vi "Update Bind RPC Template.vi"(8 "error in (no error)":errorcluster, 11 "Server Library (Library Item) in":refnum<vi>) -> (0 "error out":errorcluster, 3 "Server Library (Library Item) out":refnum<vi>)   [LabVIEW 2019, in "gRPC Template Creation Utility.lvlib"]
uses:
  gRPC Template Creation Utility.lvlib
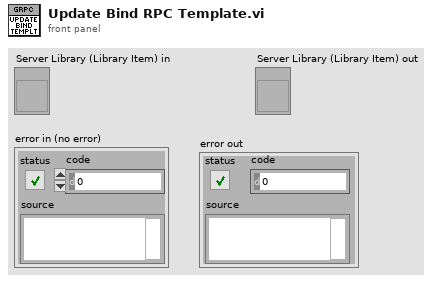
[diagram p1: front panel]
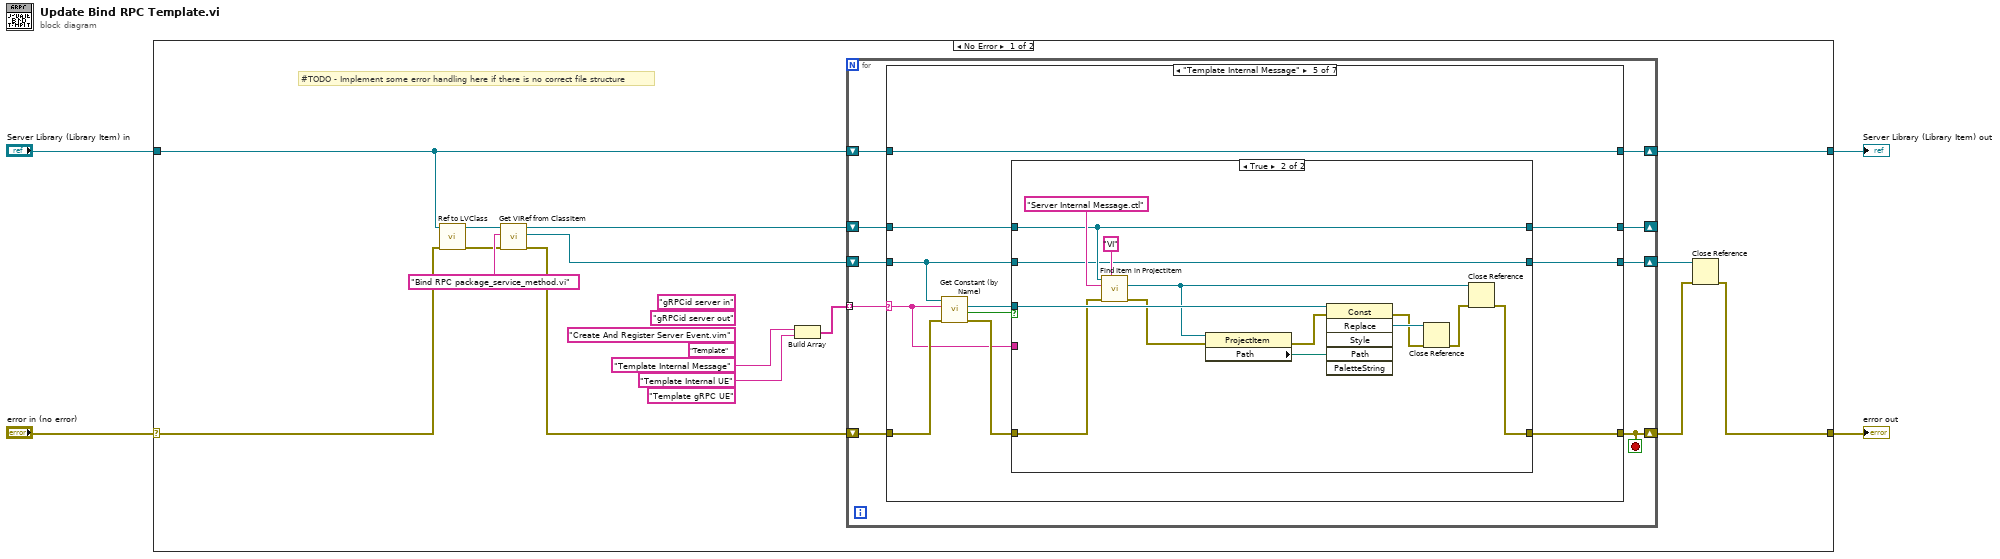
[diagram p0: block diagram]
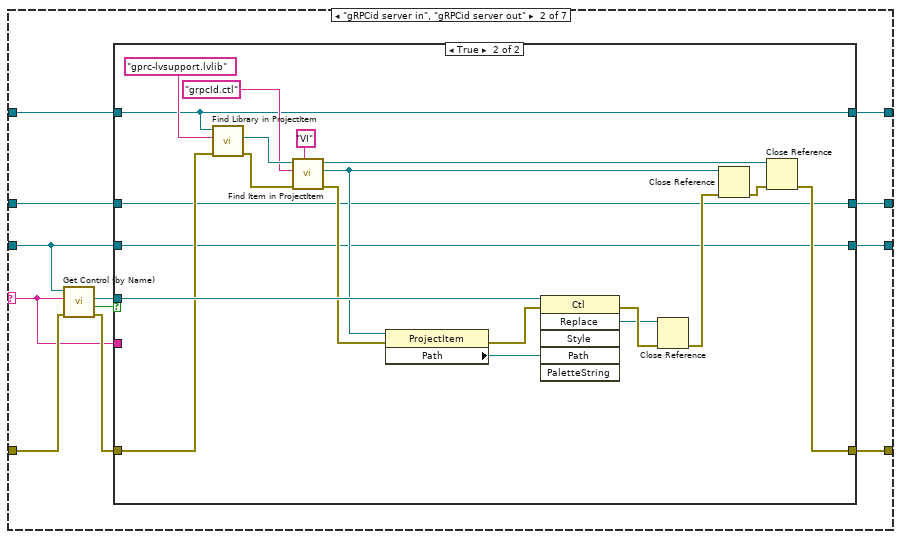
[diagram p3: hidden frame]
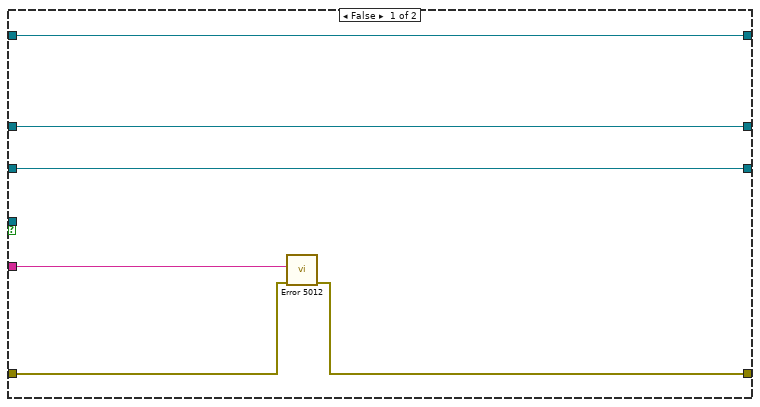
[diagram p4: hidden frame]
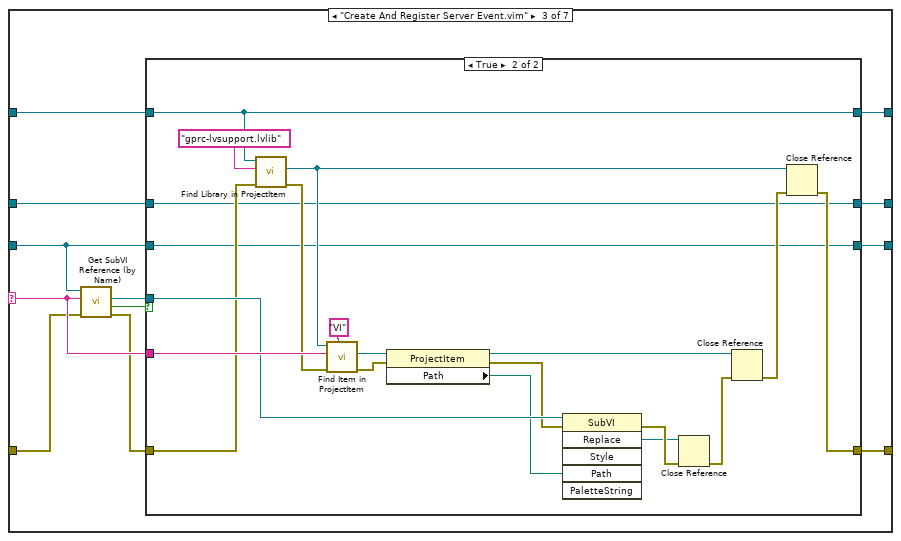
[diagram p5: hidden frame]
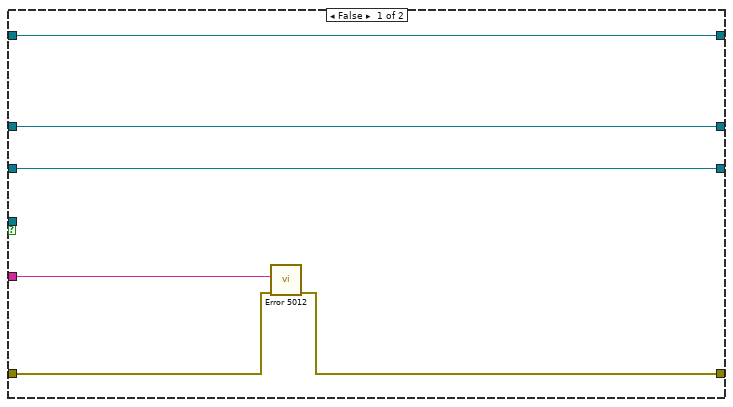
[diagram p6: hidden frame]
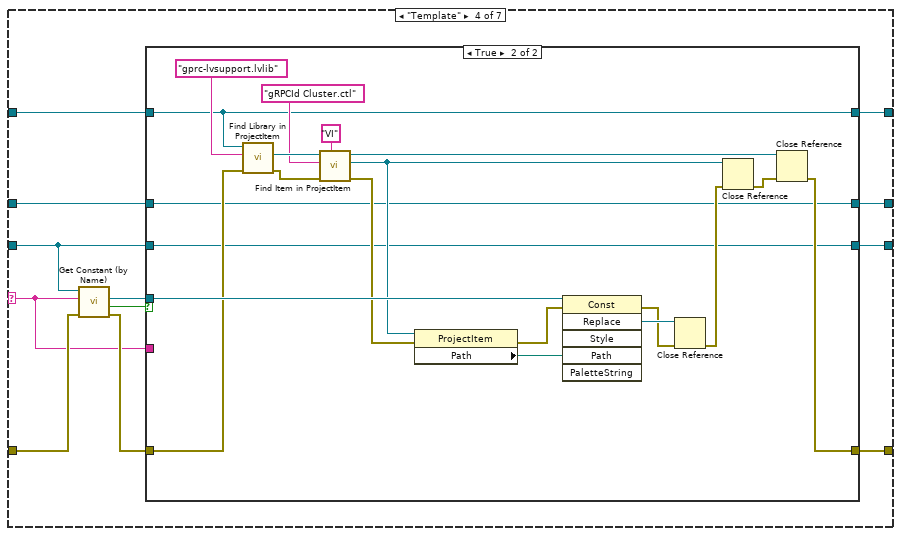
[diagram p7: hidden frame]
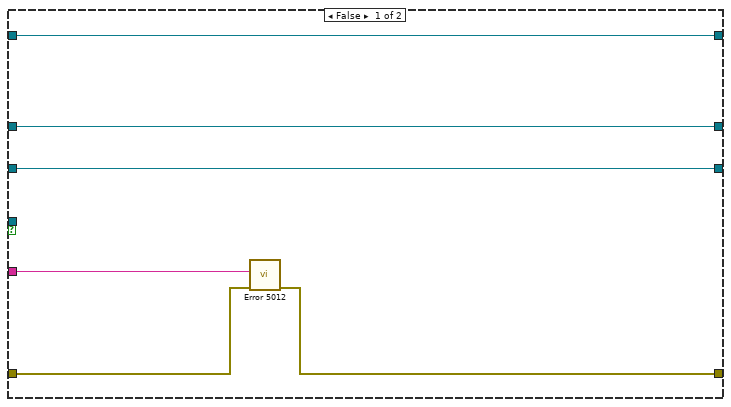
[diagram p8: hidden frame]
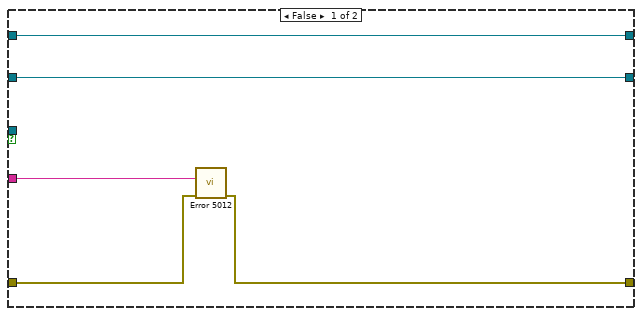
[diagram p9: hidden frame]
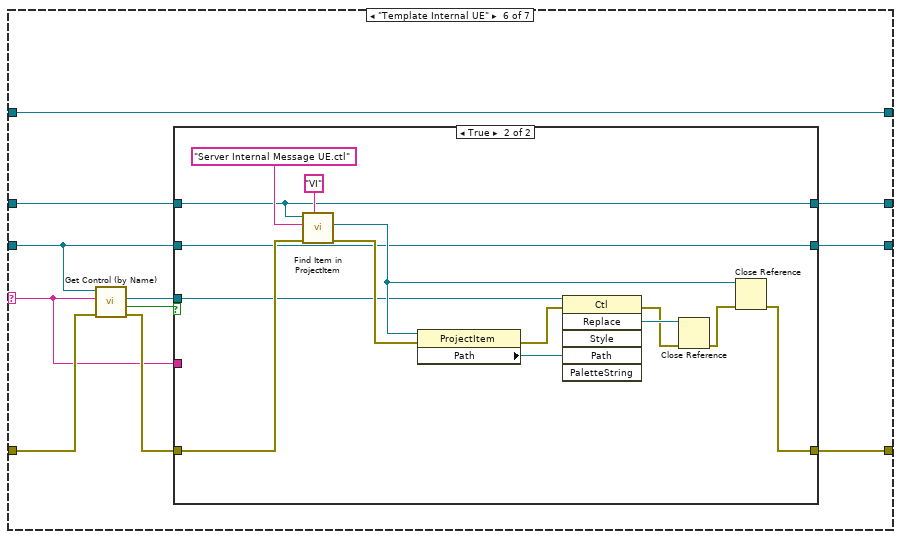
[diagram p10: hidden frame]
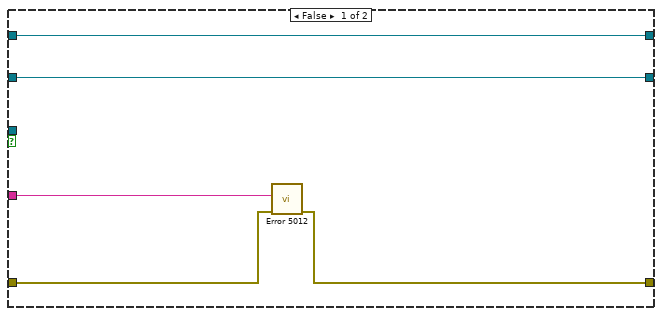
[diagram p11: hidden frame]
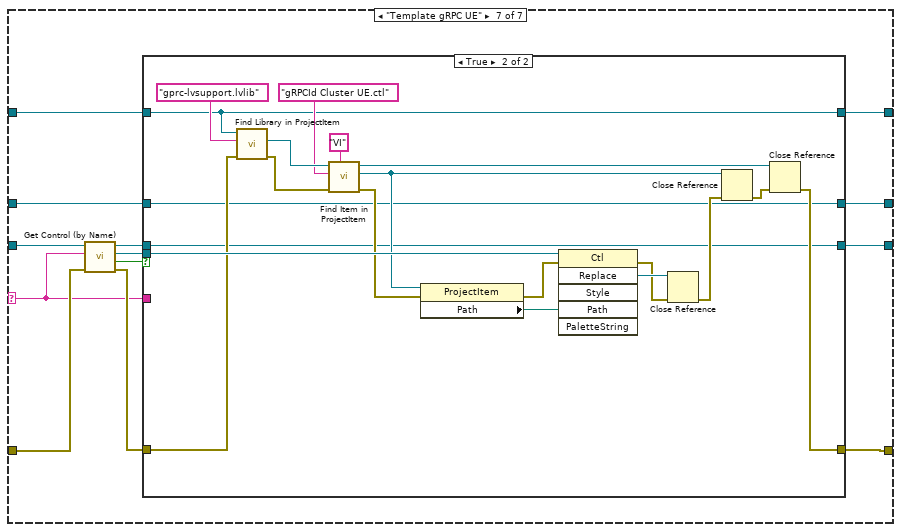
[diagram p12: hidden frame]
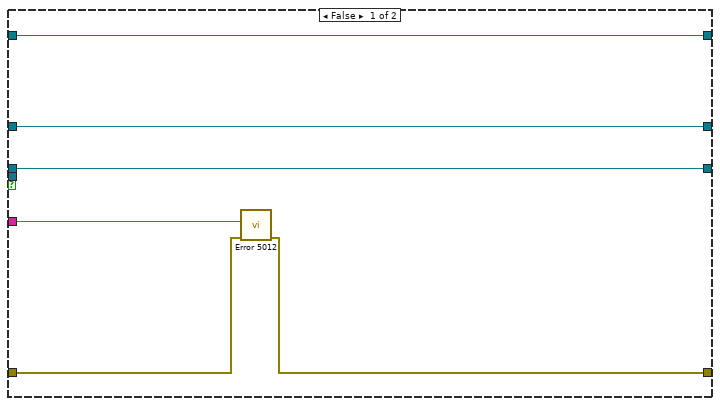
[diagram p13: hidden frame]
diagram:
  n1 = case shown="No Error" "error in (no error)" {
    selector: "error in (no error)" -> [w18 w247]
    tunnel: "Server Library (Library Item) in" -> [w5 w246]
    tunnel: [w8 w247] -> w3
    tunnel: [w11 w246] -> w1
    frame No Error {
      (unwired) "Template gRPC UE" ("Item Name")
      (unwired) "Template" ("Item Name")
      (unwired) "Create And Register Server Event.vim" ("Item Name")
      (unwired) "gRPCid server out" ("Item Name")
      (unwired) "gRPCid server in" ("Item Name")
      # "#TODO - Implement some error handling here if there is no correct file structure"
      n2 = call "Ref to LVClass.vi"("error in (no error)"=w18, "ProjectItem in"=w5) -> ("error out"=w6:errorcluster, "LVClassLibrary out"=w7:refnum<vi>)  [unwired: 8 in]
      n3 = call "Get VIRef from ClassItem.vi"("error in (no error)"=w6, "Item Name"="Bind RPC package_service_method.vi", "LVClassLibrary in"=w7) -> ("error out"=w13:errorcluster, "VIref out"=w12:refnum<vi>, "LVClassLibrary out"=w15:refnum<vi>)  [unwired: 5 in, 1 out]
      n4 = Build Array("Template Internal Message" ("Item Name"), "Template Internal UE" ("Item Name")) -> (w14:string[])
      n5 = for {
        shift-right: [w26] -> w11
        shift-left: w5 -> [w27]
        tunnel: w14 -> [w28] mode=indexing
        shift-right: [w20] -> w9
        shift-left: w13 -> [w25]
        shift-right: [w22] -> _
        shift-left: w15 -> [w23]
        shift-right: [w21] -> w10
        shift-left: w12 -> [w24]
        stop <- w20 stop-if-true
        n6 = case shown="\"Template Internal Message\"" w28 {
          selector: w28 -> [_ w33 w81 w109 w147 w177 w207]
          tunnel: w27 -> [w32 w44 w82 w120 w157 w187 w216]
          tunnel: [w32 w34 w71 w110 w157 w187 w212] -> w26
          tunnel: w24 -> [w29 w38 w75 w114 w149 w180 w219]
          tunnel: w25 -> [w31 w42 w79 w118 w155 w185 w218]
          tunnel: [w31 w40 w77 w116 w154 w186 w214] -> w20
          tunnel: w23 -> [w30 w36 w73 w112 w152 w182 w211]
          tunnel: [w30 w35 w72 w111 w150 w178 w210] -> w22
          tunnel: [w29 w37 w74 w113 w148 w179 w208] -> w21
          frame "None", Default {
          }
          frame "gRPCid server in", "gRPCid server out" {
            n7 = call "Get Control (by Name).vi"("error in (no error)"=w42, "Control Label"=w33, "Owner VI in"=w38) -> ("error out"=w41:errorcluster, "Found ?"=w39:bool, "Control Refnum"=w43:refnum<vi>)  [unwired: 5 in, 1 out]
            n8 = case shown="True" w39 {
              tunnel: w44 -> [w50 w51]
              tunnel: w43 -> [_ w66]
              tunnel: w41 -> [w47 w64]
              tunnel: [w45 w54] -> w40
              tunnel: w38 -> [w48 w53]
              tunnel: [w48 w53] -> w37
              tunnel: w36 -> [w49 w52]
              tunnel: [w49 w52] -> w35
              tunnel: [w50 w51] -> w34
              tunnel: w33 -> [w46 _]
              frame False {
                n9 = call "Error 5012.vi"("error in (no error)"=w47, "Element Name"=w46) -> ("error out"=w45:errorcluster)  [unwired: 9 in]
              }
              frame True {
                n10 = call "Find Library in ProjectItem.vi"("error in (no error)"=w64, "Library Name"="gprc-lvsupport.lvlib", "ProjectItem in"=w51) -> ("error out"=w63:errorcluster, "Library out"=w69:refnum<vi>)  [unwired: 5 in, 2 out]
                n11 = call "Find Item in ProjectItem.vi"("Item Type"="VI", "error in (no error)"=w63, "Name"="grpcId.ctl", "ProjectItem in"=w69) -> ("error out"=w62:errorcluster, "Item Refnum out"=w57:refnum<vi>, "ProjectItem out"=w55:refnum<vi>)  [unwired: 4 in, 1 out]
                n12 = property class="ProjectItem"(reference=w57, error in=w62) -> (error out=w59:errorcluster, "Path"=w65:path)  [unwired: 1 out]
                n13 = invoke class="Ctl" method="Replace"(reference=w66, error in=w59, "Path"=w65) -> (error out=w61:errorcluster, "Replace"=w60:refnum<vi>)  [unwired: 3 in, 4 out]
                n14 = Close Reference(reference=w60, error in (no error)=w61) -> (error out=w58:errorcluster)
                n15 = Close Reference(reference=w57, error in (no error)=w58) -> (error out=w56:errorcluster)
                n16 = Close Reference(reference=w55, error in (no error)=w56) -> (error out=w54:errorcluster)
              }
            }
          }
          frame "Create And Register Server Event.vim" {
            n17 = call "Get SubVI Reference (by Name).vi"("error in (no error)"=w79, "SubVI Name"=w81, "Owner VI in"=w75) -> ("error out"=w78:errorcluster, "Found ?"=w76:bool, "SubVI Refnum out"=w80:refnum<vi>)  [unwired: 5 in, 1 out]
            n18 = case shown="True" w76 {
              tunnel: w82 -> [w88 w89]
              tunnel: w81 -> [w84 w106]
              tunnel: w80 -> [_ w105]
              tunnel: w78 -> [w85 w100]
              tunnel: [w83 w92] -> w77
              tunnel: w75 -> [w86 w91]
              tunnel: [w86 w91] -> w74
              tunnel: w73 -> [w87 w90]
              tunnel: [w87 w90] -> w72
              tunnel: [w88 w89] -> w71
              frame False {
                n19 = call "Error 5012.vi"("error in (no error)"=w85, "Element Name"=w84) -> ("error out"=w83:errorcluster)  [unwired: 9 in]
              }
              frame True {
                n20 = call "Find Library in ProjectItem.vi"("error in (no error)"=w100, "Library Name"="gprc-lvsupport.lvlib", "ProjectItem in"=w89) -> ("error out"=w99:errorcluster, "Library out"=w94:refnum<vi>)  [unwired: 5 in, 2 out]
                n21 = call "Find Item in ProjectItem.vi"("Item Type"="VI", "error in (no error)"=w99, "Name"=w106, "ProjectItem in"=w94) -> ("error out"=w98:errorcluster, "Item Refnum out"=w104:refnum<vi>)  [unwired: 4 in, 2 out]
                n22 = property class="ProjectItem"(reference=w104, error in=w98) -> (reference out=w96:refnum<vi>, error out=w97:errorcluster, "Path"=w103:path)
                n23 = invoke class="SubVI" method="Replace"(reference=w105, error in=w97, "Path"=w103) -> (error out=w102:errorcluster, "Replace"=w101:refnum<vi>)  [unwired: 3 in, 4 out]
                n24 = Close Reference(reference=w101, error in (no error)=w102) -> (error out=w95:errorcluster)
                n25 = Close Reference(reference=w96, error in (no error)=w95) -> (error out=w93:errorcluster)
                n26 = Close Reference(reference=w94, error in (no error)=w93) -> (error out=w92:errorcluster)
              }
            }
          }
          frame "Template" {
            n27 = call "Get Constant (by Name).vi"("error in (no error)"=w118, "Constant Label"=w109, "Owner VI in"=w114) -> ("error out"=w117:errorcluster, "Found ?"=w115:bool, "Const ref out"=w119:refnum<vi>)  [unwired: 5 in, 1 out]
            n28 = case shown="True" w115 {
              tunnel: w120 -> [w126 w127]
              tunnel: w119 -> [_ w140]
              tunnel: w117 -> [w122 w133]
              tunnel: [w121 w130] -> w116
              tunnel: w114 -> [w124 w129]
              tunnel: [w124 w129] -> w113
              tunnel: w112 -> [w125 w128]
              tunnel: [w125 w128] -> w111
              tunnel: [w126 w127] -> w110
              tunnel: w109 -> [w123 _]
              frame False {
                n29 = call "Error 5012.vi"("error in (no error)"=w122, "Element Name"=w123) -> ("error out"=w121:errorcluster)  [unwired: 9 in]
              }
              frame True {
                n30 = call "Find Library in ProjectItem.vi"("error in (no error)"=w133, "Library Name"="gprc-lvsupport.lvlib", "ProjectItem in"=w127) -> ("error out"=w132:errorcluster, "Library out"=w145:refnum<vi>)  [unwired: 5 in, 2 out]
                n31 = call "Find Item in ProjectItem.vi"("Item Type"="VI", "error in (no error)"=w132, "Name"="gRPCId Cluster.ctl", "ProjectItem in"=w145) -> ("error out"=w131:errorcluster, "Item Refnum out"=w137:refnum<vi>, "ProjectItem out"=w135:refnum<vi>)  [unwired: 4 in, 1 out]
                n32 = property class="ProjectItem"(reference=w137, error in=w131) -> (error out=w141:errorcluster, "Path"=w142:path)  [unwired: 1 out]
                n33 = invoke class="Const" method="Replace"(reference=w140, error in=w141, "Path"=w142) -> (error out=w138:errorcluster, "Replace"=w139:refnum<vi>)  [unwired: 3 in, 4 out]
                n34 = Close Reference(reference=w139, error in (no error)=w138) -> (error out=w136:errorcluster)
                n35 = Close Reference(reference=w137, error in (no error)=w136) -> (error out=w134:errorcluster)
                n36 = Close Reference(reference=w135, error in (no error)=w134) -> (error out=w130:errorcluster)
              }
            }
          }
          frame "Template Internal Message" {
            n37 = call "Get Constant (by Name).vi"("error in (no error)"=w155, "Constant Label"=w147, "Owner VI in"=w149) -> ("error out"=w153:errorcluster, "Found ?"=w151:bool, "Const ref out"=w156:refnum<vi>)  [unwired: 5 in, 1 out]
            n38 = case shown="True" w151 {
              tunnel: w156 -> [_ w172]
              tunnel: [w158 w166] -> w154
              tunnel: w153 -> [w159 w165]
              tunnel: w152 -> [w162 w164]
              tunnel: [w162 w164] -> w150
              tunnel: w149 -> [w161 w163]
              tunnel: [w161 w163] -> w148
              tunnel: w147 -> [w160 _]
              frame False {
                n39 = call "Error 5012.vi"("error in (no error)"=w159, "Element Name"=w160) -> ("error out"=w158:errorcluster)  [unwired: 9 in]
              }
              frame True {
                n40 = call "Find Item in ProjectItem.vi"("Item Type"="VI", "error in (no error)"=w165, "Name"="Server Internal Message.ctl", "ProjectItem in"=w164) -> ("error out"=w167:errorcluster, "Item Refnum out"=w169:refnum<vi>)  [unwired: 4 in, 2 out]
                n41 = property class="ProjectItem"(reference=w169, error in=w167) -> (error out=w173:errorcluster, "Path"=w174:path)  [unwired: 1 out]
                n42 = invoke class="Const" method="Replace"(reference=w172, error in=w173, "Path"=w174) -> (error out=w170:errorcluster, "Replace"=w171:refnum<vi>)  [unwired: 3 in, 4 out]
                n43 = Close Reference(reference=w171, error in (no error)=w170) -> (error out=w168:errorcluster)
                n44 = Close Reference(reference=w169, error in (no error)=w168) -> (error out=w166:errorcluster)
              }
            }
          }
          frame "Template Internal UE" {
            n45 = call "Get Control (by Name).vi"("error in (no error)"=w185, "Control Label"=w177, "Owner VI in"=w180) -> ("error out"=w184:errorcluster, "Found ?"=w181:bool, "Control Refnum"=w183:refnum<vi>)  [unwired: 5 in, 1 out]
            n46 = case shown="True" w181 {
              tunnel: [w189 w197] -> w186
              tunnel: w184 -> [w190 w196]
              tunnel: w183 -> [_ w195]
              tunnel: w182 -> [w192 w193]
              tunnel: w180 -> [w191 w194]
              tunnel: [w191 w194] -> w179
              tunnel: [w192 w193] -> w178
              tunnel: w177 -> [w188 _]
              frame False {
                n47 = call "Error 5012.vi"("error in (no error)"=w190, "Element Name"=w188) -> ("error out"=w189:errorcluster)  [unwired: 9 in]
              }
              frame True {
                n48 = call "Find Item in ProjectItem.vi"("Item Type"="VI", "error in (no error)"=w196, "Name"="Server Internal Message UE.ctl", "ProjectItem in"=w193) -> ("error out"=w198:errorcluster, "Item Refnum out"=w200:refnum<vi>)  [unwired: 4 in, 2 out]
                n49 = property class="ProjectItem"(reference=w200, error in=w198) -> (error out=w203:errorcluster, "Path"=w204:path)  [unwired: 1 out]
                n50 = invoke class="Ctl" method="Replace"(reference=w195, error in=w203, "Path"=w204) -> (error out=w201:errorcluster, "Replace"=w202:refnum<vi>)  [unwired: 3 in, 4 out]
                n51 = Close Reference(reference=w202, error in (no error)=w201) -> (error out=w199:errorcluster)
                n52 = Close Reference(reference=w200, error in (no error)=w199) -> (error out=w197:errorcluster)
              }
            }
          }
          frame "Template gRPC UE" {
            n53 = call "Get Control (by Name).vi"("error in (no error)"=w218, "Control Label"=w207, "Owner VI in"=w219) -> ("error out"=w215:errorcluster, "Found ?"=w213:bool, "Control Refnum"=w217:refnum<vi>, "Owner VI out"=w209:refnum<vi>)  [unwired: 5 in]
            n54 = case shown="True" w213 {
              tunnel: w217 -> [_ w240]
              tunnel: w216 -> [w225 w228]
              tunnel: w215 -> [w222 w234]
              tunnel: [w220 w229] -> w214
              tunnel: [w225 w228] -> w212
              tunnel: w211 -> [w224 w227]
              tunnel: [w224 w227] -> w210
              tunnel: w209 -> [w223 w226]
              tunnel: [w223 w226] -> w208
              tunnel: w207 -> [w221 _]
              frame False {
                n55 = call "Error 5012.vi"("error in (no error)"=w222, "Element Name"=w221) -> ("error out"=w220:errorcluster)  [unwired: 9 in]
              }
              frame True {
                n56 = call "Find Library in ProjectItem.vi"("error in (no error)"=w234, "Library Name"="gprc-lvsupport.lvlib", "ProjectItem in"=w228) -> ("error out"=w235:errorcluster, "Library out"=w238:refnum<vi>)  [unwired: 5 in, 2 out]
                n57 = call "Find Item in ProjectItem.vi"("Item Type"="VI", "error in (no error)"=w235, "Name"="gRPCId Cluster UE.ctl", "ProjectItem in"=w238) -> ("error out"=w233:errorcluster, "Item Refnum out"=w232:refnum<vi>, "ProjectItem out"=w231:refnum<vi>)  [unwired: 4 in, 1 out]
                n58 = property class="ProjectItem"(reference=w232, error in=w233) -> (error out=w244:errorcluster, "Path"=w245:path)  [unwired: 1 out]
                n59 = invoke class="Ctl" method="Replace"(reference=w240, error in=w244, "Path"=w245) -> (error out=w242:errorcluster, "Replace"=w243:refnum<vi>)  [unwired: 3 in, 4 out]
                n60 = Close Reference(reference=w243, error in (no error)=w242) -> (error out=w241:errorcluster)
                n61 = Close Reference(reference=w232, error in (no error)=w241) -> (error out=w230:errorcluster)
                n62 = Close Reference(reference=w231, error in (no error)=w230) -> (error out=w229:errorcluster)
              }
            }
          }
        }
      }
      n63 = Close Reference(reference=w10, error in (no error)=w9) -> (error out=w8:errorcluster)
    }
    frame Error {
    }
  }
  "error out" <- w3
  "Server Library (Library Item) out" <- w1
